vi "WriteJointPositionRegister.vi"(8 "Value":dbl[](array[numeric]), 9 "index":i32, 10 "Snpx":refnum<k24>, 11 "error in":errorcluster) -> (3 "error out":errorcluster)   [LabVIEW 2018, in "UnderAutomation.Fanuc.lvlib"]
uses:
  UnderAutomation.Fanuc.lvlib
  C:/Users/fg/Documents/Fanuc.vi/LabVIEW_2024/UnderAutomation.Fanuc/lib/UnderAutomation.Fanuc.dll
  LabVIEW_2024/UnderAutomation.Fanuc/lib/UnderAutomation.Fanuc.dll
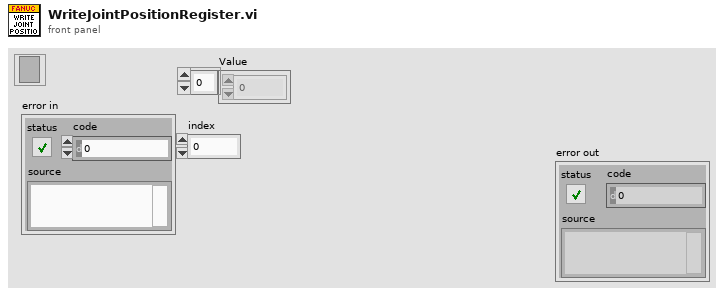
[diagram p1: front panel]
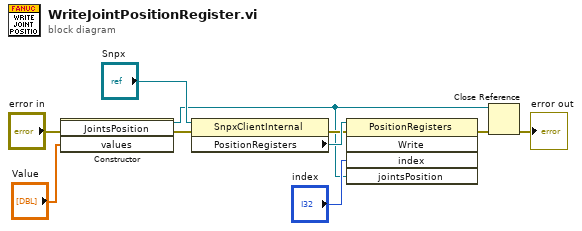
[diagram p0: block diagram]
diagram:
  n1 = constructor class="JointsPosition"(error in="error in", "values"="Value") -> (reference out=w1:refnum<k24>, error out=w2:errorcluster)  [unwired: 2 in, 2 out]
  n2 = property class="SnpxClientInternal"(reference="Snpx", error in=w2) -> (error out=w8:errorcluster, "PositionRegisters"=w9:refnum<k24>)  [unwired: 1 out]
  n3 = invoke class="PositionRegisters" method="Write"(reference=w9, error in=w8, "index"="index", "jointsPosition"=w1) -> (error out=w6:errorcluster)  [unwired: 1 in, 4 out]
  n4 = Close Reference(reference=w1, error in (no error)=w6) -> (error out=→"error out":errorcluster)
